vi "Destroy Signals Wrapper.vi"   [LabVIEW 2015]
uses:
  <vilib>/LV-Signals/destroy-xnode/LV-Destroy-Signals.xnode
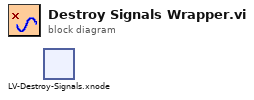
[diagram p0: block diagram]
diagram:
  n1 = xnode "LV-Destroy-Signals.xnode"() -> ()  [unwired: 2 in, 2 out]
